vi "debug.vi"(8 "error in (no error)":errorcluster, 11 "Message":string) -> ()   [LabVIEW 2017]
uses:
  <vilib>/NI Veristand/Custom Device Tools/Custom Device Utility Library/RT Debug String Color Spec.ctl
  <vilib>/NI VeriStand/Custom Device Tools/Custom Device Utility Library/Custom Device Utility Library.lvlib
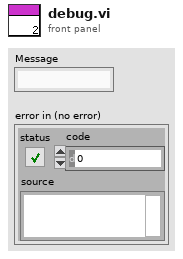
[diagram p1: front panel]
types:
  T1 = typedef "Custom Device Utility Library.lvlib/RT Debug String Color Spec.ctl" = u16
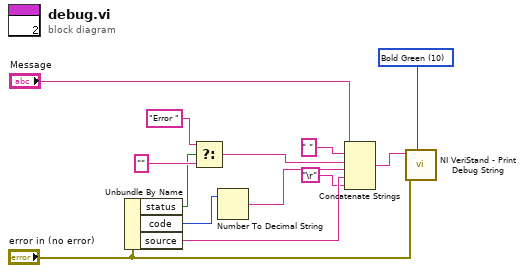
[diagram p0: block diagram]
diagram:
  w3 = T1 10 items=["Plain White"=7, "Bold White"=15, "Bold Blue"=9, "Bold Green"=10, "Bold Red"=12] ("Attribute")
  n1 = Unbundle By Name("error in (no error)") -> ("status"=w8:bool, "code"=w7:i32, "source"=w6:string)
  n2 = Select(t="Error " ("Message"), s=w8, f="" ("Message")) -> (s? t:f=w4:string)
  n3 = Number To Decimal String(number=w7) -> (decimal integer string=w5:string)  [unwired: 1 in]
  n4 = Concatenate Strings("Message", " " ("string"), w4, w5, w6, "\r") -> (w12:string)
  n5 = call <vilib>:"NI VeriStand - Print Debug String.vi"("Attribute"=w3, "error in (no error)"="error in (no error)", "Message"=w12) -> ()  [unwired: 8 in, 1 out]
